vi "ConvertTo(waveforms).vi"(8 "error in":errorcluster, 9 "Message Payload":variant) -> (0 "error out":errorcluster, 1 "Message Payload  waveforms":waveform(dbl)[](array[waveform]))   [LabVIEW 2017]
doc: "Convert variant to DAQmx waveform type array\n\nBolder Software LLC"
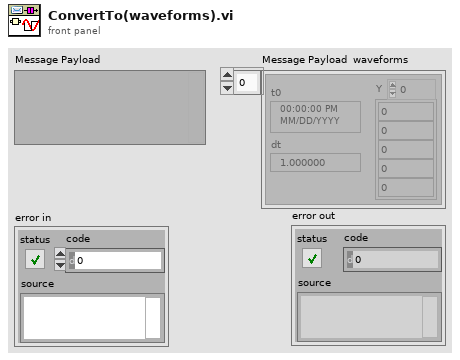
[diagram p1: front panel]
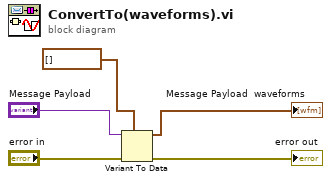
[diagram p0: block diagram]
diagram:
  n1 = Variant To Data(error in="error in", type=waveform(dbl)[] [], Variant="Message Payload") -> (data=→"Message Payload  waveforms":waveform(dbl)[], error out=→"error out":errorcluster)
